vi "speedscalc.vi"() -> ()   [LabVIEW 2015]
uses:
  <vilib>/Utility/file.llb/Write Delimited Spreadsheet (DBL).vi
panel:
  in  "Min Velocity":i32
  in  "Max Velocity":i32
  in  "Angle":dbl
  in  "Framerate":i32
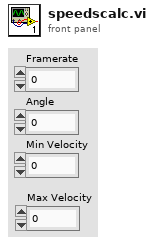
[diagram p1: front panel]
types:
  T1 = cluster{"Firing Angle":dbl, "Framerate":dbl, "Initial Velocity":dbl}
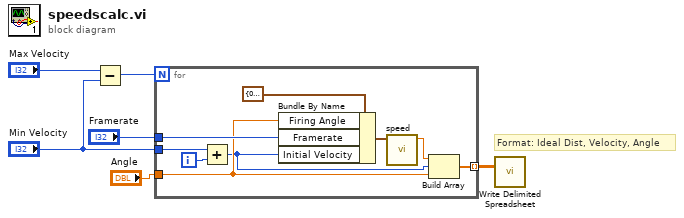
[diagram p0: block diagram]
diagram:
  # "Format: Ideal Dist, Velocity, Angle"
  n1 = Subtract(x="Max Velocity", y="Min Velocity") -> (x-y=w5:i32)
  n2 = for {
    N: w5 -> [_]
    tunnel: "Min Velocity" -> [w15]
    tunnel: "Framerate" -> [w12]
    tunnel: "Angle" -> [w10]
    tunnel: [w11] -> w1 mode=indexing
    i -> [w14]
    n3 = Add(x=w15, y=w14) -> (x+y=w9:i32)
    n4 = Bundle By Name(cluster=T1 {"Firing Angle"=0.0, "Framerate"=0.0, "Initial Velocity"=0.0} ("Parameters"), "Firing Angle"=w10, "Framerate"=w12, "Initial Velocity"=w9) -> (w8:T1)
    n5 = call "speed.vi"("Parameters"=w8) -> ("Distance"=w7:dbl)  [unwired: 10 in]
    n6 = Build Array(w7, w9, w10) -> (w11:dbl[])
  }
  n7 = call-poly <vilib>:"Write Delimited Spreadsheet.vi"("2D data"=w1) -> ()  [unwired: 13 in, 2 out]
